vi "Read First_.vi"(8 "error in (no error)":errorcluster, 11 "BCAdmin in":refnum<class "BCAdmin.lvclass">) -> (0 "error out":errorcluster, 2 "First?":bool, 3 "BCAdmin out":refnum<class "BCAdmin.lvclass">)   [LabVIEW 2017, in "BusController.lvlib" / "BCAdmin.lvclass"]
uses:
  BCAdmin.lvclass
  BCAdmin.lvclass/BCAdmin.ctl
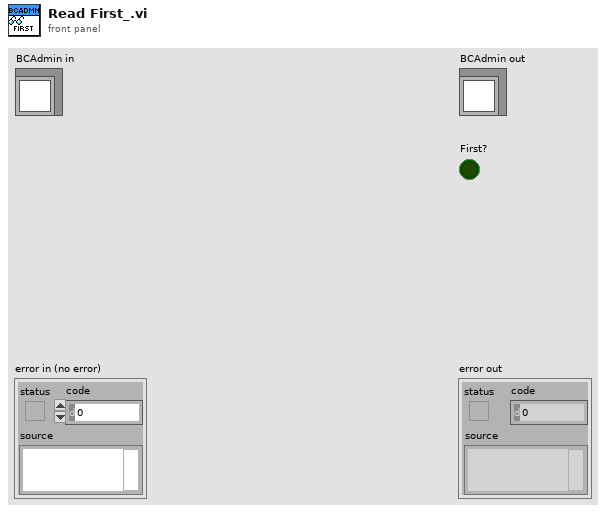
[diagram p1: front panel]
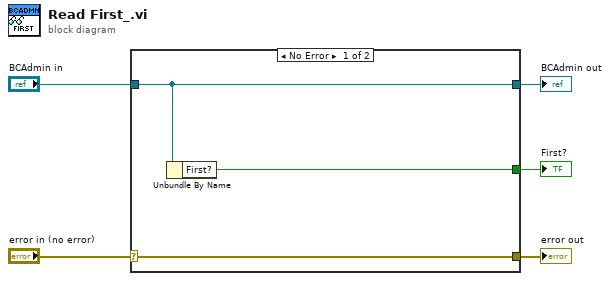
[diagram p0: block diagram]
diagram:
  n1 = case shown="No Error" "error in (no error)" {
    selector: "error in (no error)" -> [w8 w9]
    tunnel: [w8 w9] -> w4
    tunnel: [w7 w10] -> w2
    tunnel: "BCAdmin in" -> [w7 w10]
    tunnel: [w6 _] -> w1
    frame No Error {
      n2 = Unbundle By Name(w7) -> ("First?"=w6:bool)
    }
    frame Error {
    }
  }
  "error out" <- w4
  "BCAdmin out" <- w2
  "First?" <- w1
